vi "time2mm.vi"(2 "Offset (mm)":dbl, 3 "time":dbl) -> (0 "position (mm)":dbl)   [LabVIEW 2020]
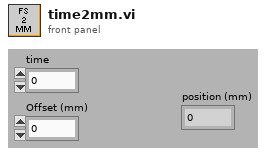
[diagram p1: front panel]
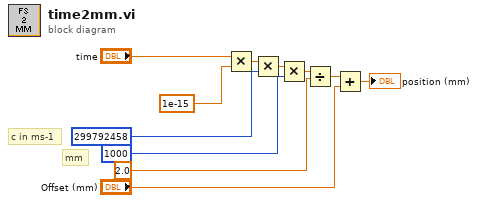
[diagram p0: block diagram]
diagram:
  # "mm"
  # "c in ms-1"
  n1 = Multiply(x="time", y=1e-15) -> (x*y=w1:dbl)
  n2 = Multiply(x=w1, y=299792458) -> (x*y=w3:dbl)
  n3 = Multiply(x=w3, y=1000) -> (x*y=w5:dbl)
  n4 = Divide(x=w5, y=2.0) -> (x/y=w8:dbl)
  n5 = Add(x=w8, y="Offset (mm)") -> (x+y=→"position (mm)":dbl)
